vi "Write Context I32.vi"(8 "error in (no error)":errorcluster, 10 "Context I32":i32, 11 "Context Actor in":refnum<class "Context Actor.lvclass">) -> (0 "error out":errorcluster, 3 "Context Actor out":refnum<class "Context Actor.lvclass">)   [LabVIEW 2021, in "Context Actor.lvlib" / "Context Actor.lvclass"]
uses:
  Context Actor.lvclass
  Context Actor.lvclass/Context Actor.ctl
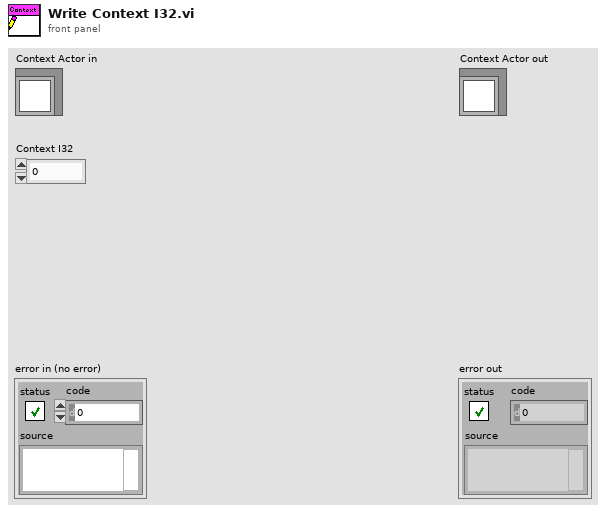
[diagram p1: front panel]
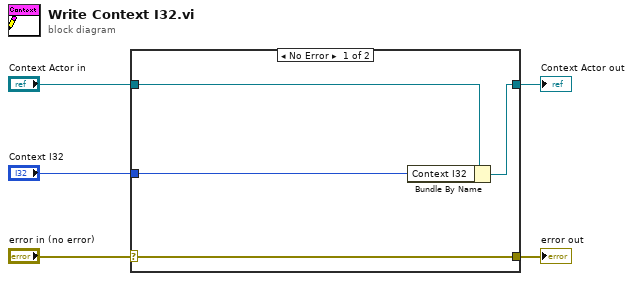
[diagram p0: block diagram]
diagram:
  n1 = case shown="No Error" "error in (no error)" {
    selector: "error in (no error)" -> [w9 w10]
    tunnel: [w9 w10] -> w4
    tunnel: [w7 w11] -> w2
    tunnel: "Context Actor in" -> [w8 w11]
    tunnel: "Context I32" -> [w6 _]
    frame No Error {
      n2 = Bundle By Name(cluster=w8, "Context I32"=w6) -> (w7:refnum<class "Context Actor.lvclass">)
    }
    frame Error {
    }
  }
  "error out" <- w4
  "Context Actor out" <- w2
